vi "RTMain.vi"() -> ()   [LabVIEW 2017]
uses:
  TypeDefs/dataOut.ctl
  TypeDefs/dataIn.ctl
  TypeDefs/UDPListenFGVCtrl.ctl
  TypeDefs/dataFGVState.ctl
panel:
  out "error out":errorcluster
  out "data in":T1
  in  "DataOut":T2
  in  "stop":bool
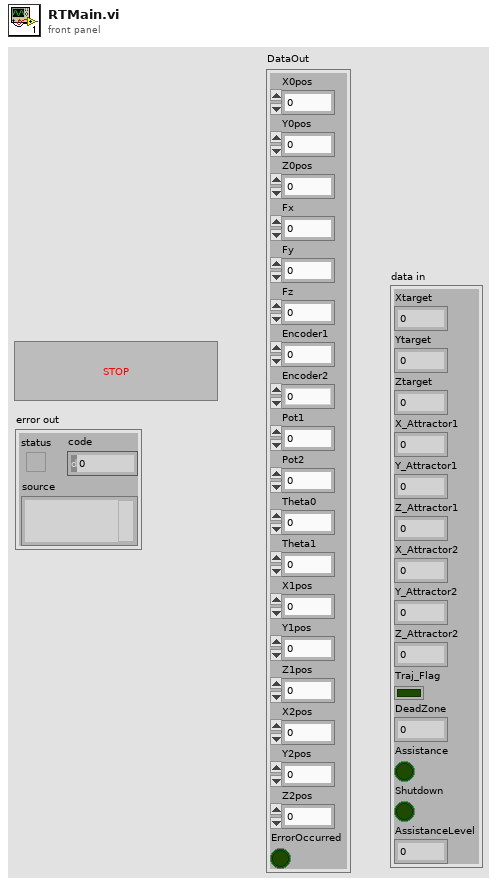
[diagram p1: front panel]
types:
  T1 = typedef "dataIn.ctl" = cluster{"Xtarget":dbl, "Ytarget":dbl, "Ztarget":dbl, "X_Attractor1":dbl, "Y_Attractor1":dbl, "Z_Attractor1":dbl, "X_Attractor2":dbl, "Y_Attractor2":dbl, "Z_Attractor2":dbl, "Traj_Flag":bool, "DeadZone":dbl, "Assistance":bool, "Shutdown":bool, "AssistanceLevel":dbl}
  T2 = typedef "dataOut.ctl" = cluster{"X0pos":dbl, "Y0pos":dbl, "Z0pos":dbl, "Fx":dbl, "Fy":dbl, "Fz":dbl, "Encoder1":i32, "Encoder2":i32, "Pot1":dbl, "Pot2":dbl, "Theta0":dbl, "Theta1":dbl, "X1pos":dbl, "Y1pos":dbl, "Z1pos":dbl, "X2pos":dbl, "Y2pos":dbl, "Z2pos":dbl, "ErrorOccurred":bool}
  T3 = typedef "UDPListenFGVCtrl.ctl" = enum16{"Read", "Write"}
  T4 = typedef "dataFGVState.ctl" = enum16{"init", "write data out", "read data out", "write data in", "read data in"}
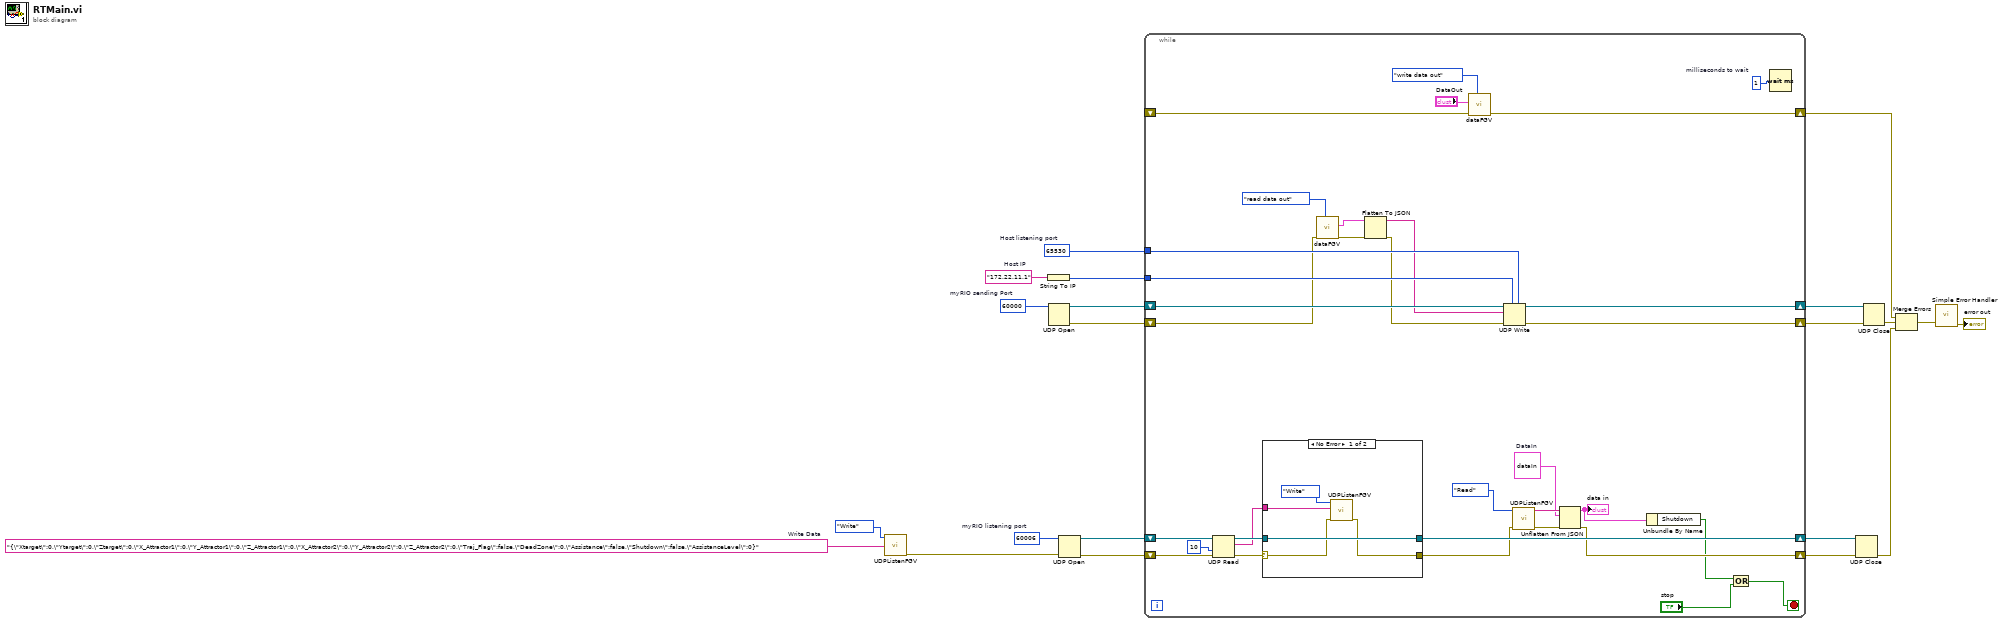
[diagram p0: block diagram]
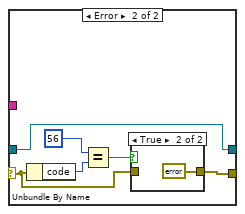
[diagram p2: hidden frame]
diagram:
  w3 = "{\"Xtarget\":0,\"Ytarget\":0,\"Ztarget\":0,\"X_Attractor1\":0,\"Y_Attractor1\":0,\"Z_Attractor1\":0,\"X_Attractor2\":0,\"Y_Attractor2\":0,\"Z_Attractor2\":0,\"Traj_Flag\":false,\"DeadZone\":0,\"Assistance\":false,\"Shutdown\":false,\"AssistanceLevel\":0}"  # Write Data
  w19 = u16 60006  # myRIO listening port
  w18 = u16 65530  # Host listening port
  w20 = "172.22.11.1"  # Host IP
  w21 = u16 60000  # myRIO sending Port
  n1 = call "UDPListenFGV.vi"("Write Data"=w3, "Enum"=UDPListenFGVCtrl."Write") -> ("error out"=w2:errorcluster)  [unwired: 8 in, 1 out]
  n2 = String To IP(1:w20) -> (0:w17:u32)
  n3 = UDP Open(11:w21) -> (port=w16:refnum<k16>, 0:w15:errorcluster)  [unwired: 4 in, 1 out]
  n4 = UDP Open(8:w2, 11:w19) -> (port=w14:refnum<k16>, 0:w13:errorcluster)  [unwired: 3 in, 1 out]
  n5 = while {
    tunnel: w18 -> [w43]
    tunnel: w17 -> [w44]
    shift-right: [w47] -> w8
    shift-left: w16 -> [w45]
    shift-right: [w46] -> w7
    shift-left: w15 -> [w34]
    shift-right: [w42] -> w10
    shift-left: w14 -> [w50]
    shift-right: [w27] -> w9
    shift-left: w13 -> [w49]
    shift-right: [w36] -> w5
    shift-left: _ -> [w37]
    stop <- w24 stop-if-true
    w26 = T1 {"Xtarget"=0.0, "Ytarget"=0.0, "Ztarget"=0.0, "X_Attractor1"=0.0, "Y_Attractor1"=0.0, "Z_Attractor1"=0.0, "X_Attractor2"=0.0, "Y_Attractor2"=0.0, "Z_Attractor2"=0.0, "Traj_Flag"=FALSE, "DeadZone"=0.0, "Assistance"=FALSE, "Shutdown"=FALSE, "AssistanceLevel"=0.0}  # DataIn
    w48 = u32 1  # milliseconds to wait
    n6 = UDP Read(connection ID=w50, timeout ms (25000)=10, 8:w49) -> (data out=w51:string, error out=w53:errorcluster, 3:w52:refnum<k16>)  [unwired: 1 in, 2 out]
    n7 = case shown="No Error" w53 {
      selector: w53 -> [w58 w61]
      tunnel: w52 -> [w59 w60]
      tunnel: w51 -> [w56 _]
      tunnel: [w57 w62] -> w41
      tunnel: [w59 w60] -> w42
      frame No Error {
        n8 = call "UDPListenFGV.vi"("error in (no error)"=w58, "Write Data"=w56, "Enum"=UDPListenFGVCtrl."Write") -> ("error out"=w57:errorcluster)  [unwired: 7 in, 1 out]
      }
      frame Error {
        n9 = Unbundle By Name(w61) -> ("code"=w65:i32)
        n10 = Equal?(x=56, y=w65) -> (x = y?=w63:bool)
        n11 = case shown="True" w63 {
          tunnel: [w66 errorcluster {"status"=FALSE, "code"=0, "source"=""} ("error constant")] -> w62
          tunnel: w61 -> [w66 _]
          frame False {
          }
          frame True {
          }
        }
      }
    }
    n12 = call "dataFGV.vi"("Enum"=dataFGVState."read data out", "error in (no error)"=w34) -> ("error out"=w32:errorcluster, "DataOut"=w33:T2)  [unwired: 7 in, 1 out]
    n13 = Flatten To JSON(anything=w33, error in (no error)=w32) -> (JSON string=w30:string, 11:w31:errorcluster)  [unwired: 1 in]
    n14 = call "dataFGV.vi"("Enum"=dataFGVState."write data out", "error in (no error)"=w37, "DataOut"="DataOut") -> ("error out"=w36:errorcluster)  [unwired: 6 in, 2 out]
    n15 = UDP Write(address=w44, port or service name=w43, connection ID=w45, data in=w30, 8:w31) -> (error out=w46:errorcluster, 3:w47:refnum<k16>)  [unwired: 1 in]
    n16 = call "UDPListenFGV.vi"("error in (no error)"=w41, "Enum"=UDPListenFGVCtrl."Read") -> ("error out"=w28:errorcluster, "Read Data"=w29:string)  [unwired: 8 in]
    n17 = Unflatten From JSON(JSON string=w29, type and defaults=w26, error in (no error)=w28) -> (value=w23:T1, error out=w27:errorcluster)  [unwired: 4 in]
    "data in" <- w23
    n18 = Unbundle By Name(w23) -> ("Shutdown"=w22:bool)
    n19 = Or(x=w22, y="stop") -> (x .or. y?=w24:bool)
    n20 = Wait (ms)(milliseconds to wait=w48) -> ()  [unwired: 1 out]
  }
  n21 = UDP Close(connection ID=w10, 8:w9) -> (error out=w11:errorcluster)  [unwired: 1 out]
  n22 = UDP Close(connection ID=w8, 8:w7) -> (error out=w12:errorcluster)  [unwired: 1 out]
  n23 = Merge Errors(w5, w12, w11) -> (w6:errorcluster)
  n24 = call <vilib>:"Simple Error Handler.vi"("error in (no error)"=w6) -> ("error out"=→"error out":errorcluster)  [unwired: 4 in, 4 out]
